vi "Save to file.vi"(8 "error in (no error)":errorcluster, 11 "Loop Data":T1) -> (0 "error out":errorcluster)   [LabVIEW 2015]
uses:
  TypDefs/Loop Data.ctl
  <vilib>/Utility/file.llb/Write Delimited Spreadsheet (DBL).vi
panel:
  out "size(s)":i32[](array[numeric])
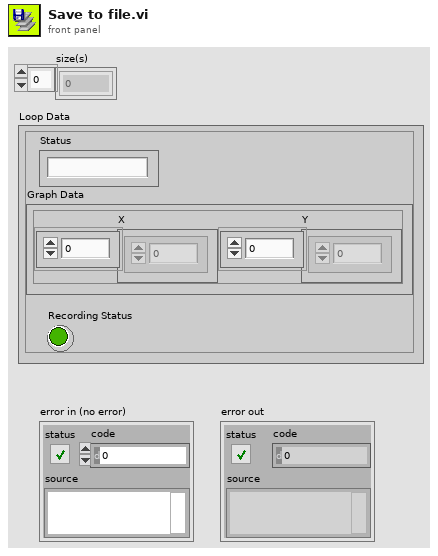
[diagram p1: front panel]
types:
  T1 = typedef "Loop Data.ctl" = cluster{"Status":string, "Graph Data":cluster{"X":dbl[], "Y":dbl[]}, "Recording Status":bool}
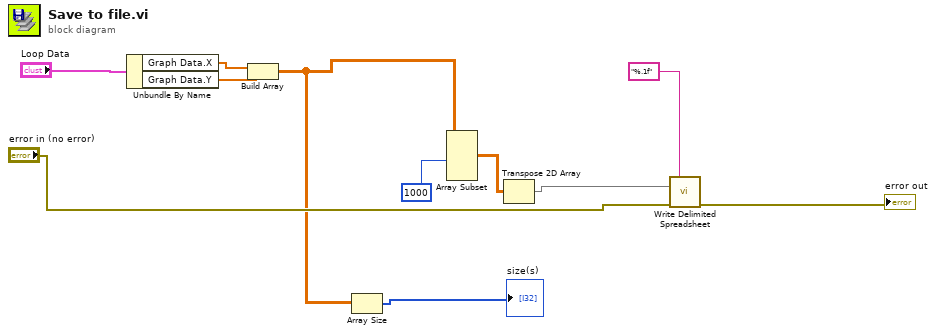
[diagram p0: block diagram]
diagram:
  n1 = Unbundle By Name("Loop Data") -> ("Graph Data.X"=w10:dbl[], "Graph Data.Y"=w9:dbl[])
  n2 = Build Array(w10, w9) -> (w2:dbl[][])
  n3 = Array Size(array=w2) -> (size(s)=→"size(s)":i32[])
  n4 = Array Subset(array=w2, length (row)=1000 ("length")) -> (w3:dbl[][])  [unwired: 3 in]
  n5 = Transpose 2D Array(2D array=w3) -> (transposed array=w8:dbl[][])
  n6 = call-poly <vilib>:"Write Delimited Spreadsheet.vi"("format (%.3f)"="%.1f", "2D data"=w8, "error in (no error)"="error in (no error)") -> ("error out"=→"error out":errorcluster)  [unwired: 11 in, 1 out]
